vi "Main.vi"() -> ()   [LabVIEW 2013]
uses:
  <vilib>/myRIO/Instrument Drivers/Onboard IO/DIO/vis/Smart Open.vi
  <vilib>/myRIO/Instrument Drivers/Onboard IO/DIO/vis/Read.vi
  <vilib>/myRIO/Common/Instrument Driver Framework/myRIO v1.0/UART/vis/myRIO v1.0 Close UART.vi
  <vilib>/myRIO/Instrument Drivers/Onboard IO/DIO/vis/Open.vi
  <vilib>/myRIO/Common/Instrument Driver Framework/myRIO v1.0/DIO/vis/myRIO v1.1 Open DIO.vi
  <vilib>/myRIO/Common/Instrument Driver Framework/myRIO v1.0/DIO/vis/myRIO v1.2 Open DIO.vi
  <vilib>/myRIO/Common/Instrument Driver Framework/Utilities/vis/Validate Channels.vi
  <vilib>/myRIO/Common/Instrument Driver Framework/myRIO v1.0/DIO/vis/myRIO v1.0 Reserve DIO.vi
  <vilib>/myRIO/Common/Instrument Driver Framework/myRIO v1.0/Resource Manager/vis/myRIO v1.0 Reserve Channel List.vi
  <vilib>/myRIO/Common/Instrument Driver Framework/myRIO v1.0/DIO/vis/myRIO v1.0 Build MUX Configuration DIO.vi
  <vilib>/myRIO/Common/Instrument Driver Framework/myRIO v1.0/Resource Manager/vis/myRIO v1.0 Reserve Channel.vi
  <vilib>/myRIO/Common/Instrument Driver Framework/myRIO v1.0/Resource Manager/vis/myRIO v1.0 Unreserve Channel.vi
  <vilib>/myRIO/Common/Instrument Driver Framework/myRIO v1.0/Resource Manager/vis/myRIO v1.0 Create Configuration List.vi
  <vilib>/myRIO/Common/Instrument Driver Framework/myRIO v1.0/Resource Manager/vis/myRIO v1.0 Build Mutex Name.vi
  <vilib>/myRIO/Common/Instrument Driver Framework/Utilities/vis/Set_Get Target Info.vi
  <vilib>/Utility/error.llb/Error Cluster From Error Code.vi
  <vilib>/myRIO/Common/Instrument Driver Framework/myRIO v1.0/myRIO v1.1 Open.vi
  <vilib>/Utility/VariantDataType/GetNumericInfo.vi
  <vilib>/myRIO/Common/Instrument Driver Framework/Utilities/vis/IO Manager.vi
  <vilib>/myRIO/Common/Instrument Driver Framework/Utilities/vis/Configuration Manager.vi
  <vilib>/myRIO/Common/Instrument Driver Framework/myRIO v1.0/Resource Manager/vis/myRIO v1.0 Configure IO.vi
  <vilib>/myRIO/Common/Instrument Driver Framework/myRIO v1.0/myRIO v1.0 Close.vi
  <vilib>/myRIO/Common/Instrument Driver Framework/myRIO v1.0/myRIO v1.2 Open.vi
  <vilib>/myRIO/Common/Instrument Driver Framework/myRIO v1.0/DIO/vis/myRIO v1.0 Read DIO.vi
  <vilib>/myRIO/Common/Instrument Driver Framework/Utilities/vis/FPGA Ref Manager.vi
  <vilib>/myRIO/Common/Instrument Driver Framework/myRIO v1.0/myRIO v1.0 Reset FPGA.vi
  <vilib>/myRIO/Instrument Drivers/Utilities/Utilities.lvlib
panel:
  out "A/DIO state":bool[](array[boolean])
  out "B/DIO state":bool[](array[boolean])
  in  "[ESC]":bool
  # "DIP switches demo"
  # "Rotary DIP"
  # "8-switch DIP"
  # "3       2       1       0"
  # "7       6       5       4       3       2       1       0"
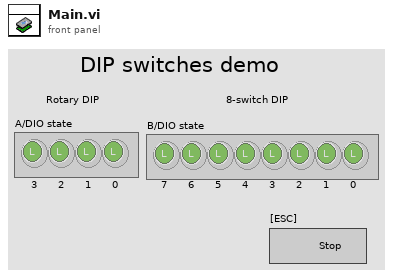
[diagram p1: front panel]
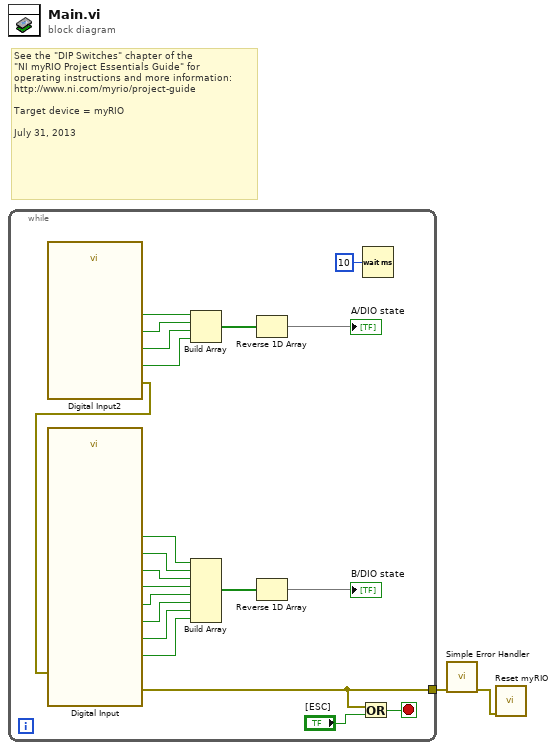
[diagram p0: block diagram]
diagram:
  # "See the \"DIP Switches\" chapter of the \n\"NI myRIO Project Essentials Guide\" for\noperating instructions and more information: \nhttp://www.ni.com/myrio/project-guide\n\nTarget device = myRIO\n\nJuly 31, 2013"
  n1 = while {
    tunnel: [w20] -> w2
    stop <- w23 stop-if-true
    n2 = call "Digital Input2"() -> ("A/DIO0 (Pin 11)"=w5:bool, "A/DIO1 (Pin 13)"=w6:bool, "A/DIO2 (Pin 15)"=w7:bool, "A/DIO3 (Pin 17)"=w8:bool, "error out"=w3:errorcluster)  [unwired: 23 in]
    n3 = call "Digital Input"("error in (no error)"=w3) -> ("B/DIO6 (Pin 23)"=w13:bool, "B/DIO7 (Pin 25)"=w12:bool, "B/DIO0 (Pin 11)"=w19:bool, "B/DIO1 (Pin 13)"=w18:bool, "B/DIO2 (Pin 15)"=w17:bool, "B/DIO3 (Pin 17)"=w16:bool, "B/DIO4 (Pin 19)"=w15:bool, "B/DIO5 (Pin 21)"=w14:bool, "error out"=w20:errorcluster)  [unwired: 18 in]
    n4 = Build Array "Build Array"(w5, w6, w7, w8) -> (w9:bool[])
    n5 = Build Array "Build Array"(w19, w18, w17, w16, w15, w14, w13, w12) -> (w11:bool[])
    n6 = Reverse 1D Array(array=w9) -> (reversed array=→"A/DIO state":bool[])
    n7 = Reverse 1D Array(array=w11) -> (reversed array=→"B/DIO state":bool[])
    n8 = Or(x=w20, y="[ESC]") -> (x .or. y?=w23:bool)
    n9 = Wait (ms)(milliseconds to wait=u32 10) -> ()  [unwired: 1 out]
  }
  n10 = call <vilib>:"Simple Error Handler.vi"("error in (no error)"=w2) -> ("error out"=w1:errorcluster)  [unwired: 4 in, 4 out]
  n11 = call <vilib>:"Reset myRIO.vi"("error in (no error)"=w1) -> ()  [unwired: 10 in, 1 out]
